vi "Serial Port Selection Select 2012 NIVerified.vi"(7 "error in (no error)":errorcluster) -> (0 "error out":errorcluster, 3 "COM Port Selected":string)   [LabVIEW 2012]
doc: "COMSelect.vi detects all instruments with an ASRL instrument name on all local and remote machines, and allows manual selection of a particular serial port. The output of this function can then be passed into a VISA Open function to generate a VISA Reference"
panel:
  in  "OK Button":bool
  in  "COM Port Selection":i32(ring) items=["ASRL1  (COM1 - Built-In)", "ASRL1  (COM1 - Communications Port)", "ASRL6  (COM6 - NI USB-232/1 SN:D2352D, Communications Port)", "ASRL10  (LPT1 - ECP Printer Port)"]
  # "Select COM Port and Press OK"
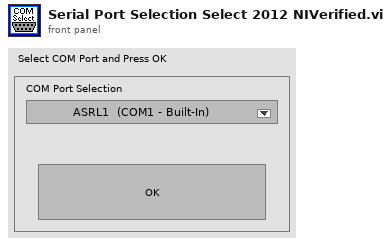
[diagram p1: front panel]
types:
  T1 = enum16{"Detect Instruments", "Open Front Panel", "Wait for User Input", "Close"}
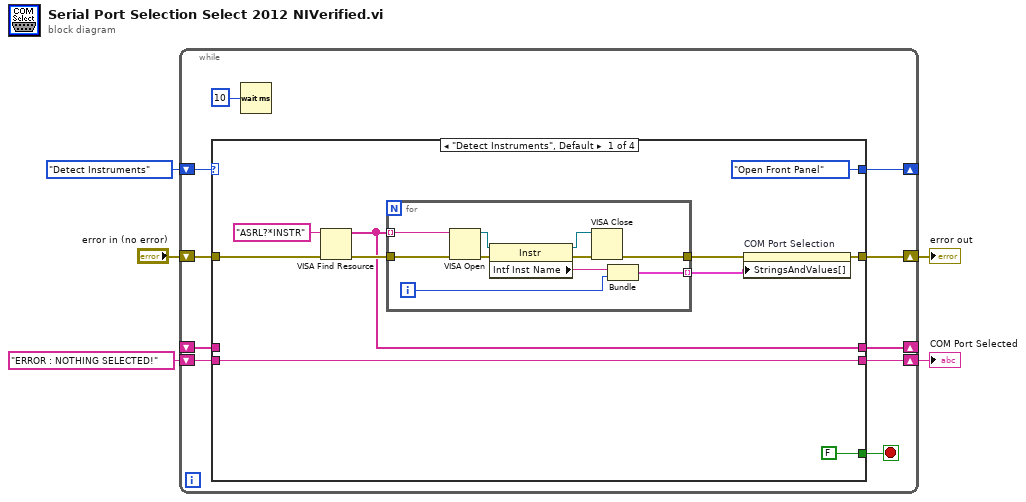
[diagram p0: block diagram]
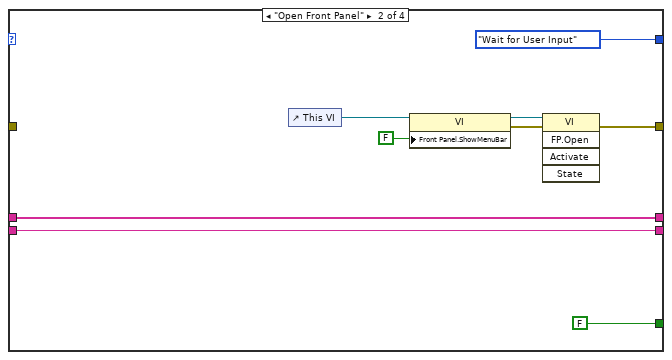
[diagram p2: hidden frame]
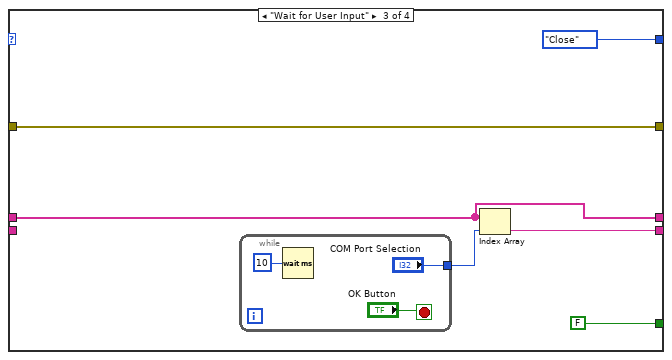
[diagram p3: hidden frame]
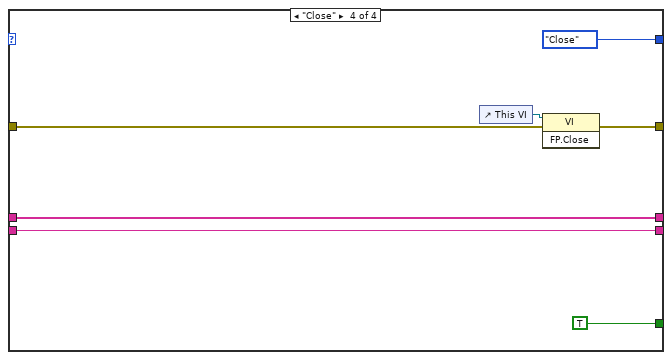
[diagram p4: hidden frame]
diagram:
  n1 = while {
    shift-right: [w14] -> _
    shift-left: T1."Detect Instruments" -> [w15]
    shift-right: [w12] -> w3
    shift-left: "error in (no error)" -> [w13]
    shift-right: [w10] -> _
    shift-left: _ -> [w9]
    shift-right: [w7] -> w2
    shift-left: "ERROR : NOTHING SELECTED!" -> [w6]
    stop <- w8 stop-if-true
    n2 = case shown="\"Detect Instruments\", Default" w15 {
      tunnel: [T1."Open Front Panel" T1."Wait for User Input" T1."Close" T1."Close"] -> w14
      tunnel: w13 -> [w21 _ w47 w55]
      tunnel: [w19 w44 w47 w54] -> w12
      tunnel: [w18 w41 w45 w58] -> w10
      tunnel: w9 -> [_ w41 w45 w58]
      tunnel: [FALSE FALSE FALSE TRUE] -> w8
      tunnel: [w16 w40 w46 w57] -> w7
      tunnel: w6 -> [w16 w40 _ w57]
      frame "Detect Instruments", Default {
        n3 = VISA Find Resource(8:w21, 11:"ASRL?*INSTR" ("expression (\"?*\")")) -> (0:w24:errorcluster, 3:w18:string[])  [unwired: 2 out]
        n4 = for {
          tunnel: w18 -> [w35] mode=indexing
          tunnel: w24 -> [w33]
          tunnel: [w28] -> w25 mode=indexing
          tunnel: [w27] -> w20
          i -> [w29]
          n5 = VISA Open(error in (no error)=w33, VISA resource name=w35) -> (VISA resource name=w34:refnum<visa-resource-name>, error out=w32:errorcluster)  [unwired: 3 out]
          n6 = property class="Instr"(reference=w34, error in=w32) -> (reference out=w30:refnum<visa-resource-name>, error out=w31:errorcluster, "Intf Inst Name"=w26:string)
          n7 = VISA Close(VISA resource name=w30, error in (no error)=w31) -> (error out=w27:errorcluster)
          n8 = Bundle("Intf Inst Name"=w26, w29) -> (w28:cluster{"Intf Inst Name":string, i32})  [unwired: 1 out]
        }
        n9 = property on="COM Port Selection" class="Ring (strict)"(error in=w20, "StringsAndValues[]"=w25) -> (error out=w19:errorcluster)  [unwired: 1 in, 1 out]
      }
      frame "Open Front Panel" {
        n10 = control-ref of="This VI"() -> (w37:refnum<vi>)
        n11 = property class="VI"(reference=w37, "Front Panel.ShowMenuBar"=FALSE ("Front Panel Window:Show Menu Bar")) -> (reference out=w38:refnum<vi>, error out=w39:errorcluster)  [unwired: 1 in]
        n12 = invoke class="VI" method="FP.Open"(reference=w38, error in=w39) -> (error out=w44:errorcluster)  [unwired: 3 in, 4 out]
      }
      frame "Wait for User Input" {
        n13 = while {
          tunnel: ["COM Port Selection"] -> w50
          stop <- "OK Button" stop-if-true
          n14 = Wait (ms)(milliseconds to wait=u32 10 ("millisecond multiple")) -> ()  [unwired: 1 out]
        }
        n15 = Index Array(array=w45, index=w50) -> (element=w46:string)
      }
      frame "Close" {
        n16 = control-ref of="This VI"() -> (w56:refnum<vi>)
        n17 = invoke class="VI" method="FP.Close"(reference=w56, error in=w55) -> (error out=w54:errorcluster)  [unwired: 1 in, 2 out]
      }
    }
    n18 = Wait (ms)(milliseconds to wait=u32 10 ("millisecond multiple")) -> ()  [unwired: 1 out]
  }
  "error out" <- w3
  "COM Port Selected" <- w2
